vi "Period.vi"(7 "Default (10)":i64=10, 11 "Sequence Config in":refnum<class "Sequence Config.lvclass">) -> (2 "Period":i64, 3 "Sequence Config out":refnum<class "Sequence Config.lvclass">)   [LabVIEW 2020, in "VolatusSeqConfig.lvlib" / "Sequence Config.lvclass"]
uses:
  Sequence Config.lvclass
  Sequence Config.lvclass/Sequence Config.ctl
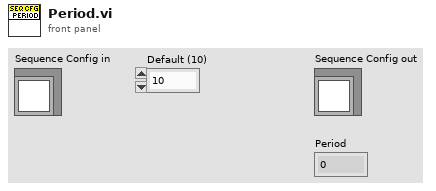
[diagram p1: front panel]
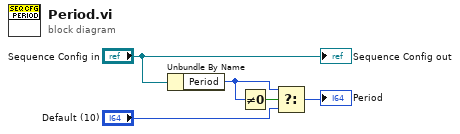
[diagram p0: block diagram]
diagram:
  n1 = Unbundle By Name("Sequence Config in") -> ("Period"=w3:i64)
  n2 = Not Equal To 0?(x=w3) -> (x != 0?=w4:bool)
  n3 = Select(t=w3, s=w4, f="Default (10)") -> (s? t:f=→"Period":i64)
  "Sequence Config out" <- "Sequence Config in"
